vi "ObtainSMQueue.vi"(8 "ErrorArray In":errorcluster[](array[cluster]), 10 "BusNumber":u8) -> (0 "ErrorArray Out":errorcluster[](array[cluster]), 3 "QueRef":T1)   [LabVIEW 2014, in "Bus.lvlib" / "NISTBus.lvclass"]
uses:
  NISTBus.lvclass
  Framework/MsgQueue/TypeDef/QueRef.ctl
  Framework/MsgQueue/TypeDef/MsgQueue.ctl
  SMQueue.ctl
  <userlib>/NIST/NISTErrorLib/NISTErrorLib.lvlib
  Framework/TestFramework.lvlib
panel:
  out "Queue Name":string
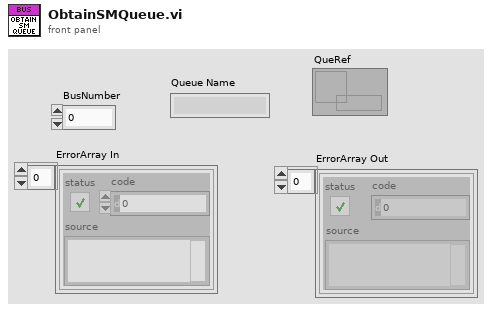
[diagram p1: front panel]
types:
  T1 = typedef "TestFramework.lvlib/QueRef.ctl" = refnum<queue>
  T2 = typedef "Bus.lvlib/NISTBus.lvclass/SMQueue.ctl" = cluster{"Msg":string, "Data":variant}
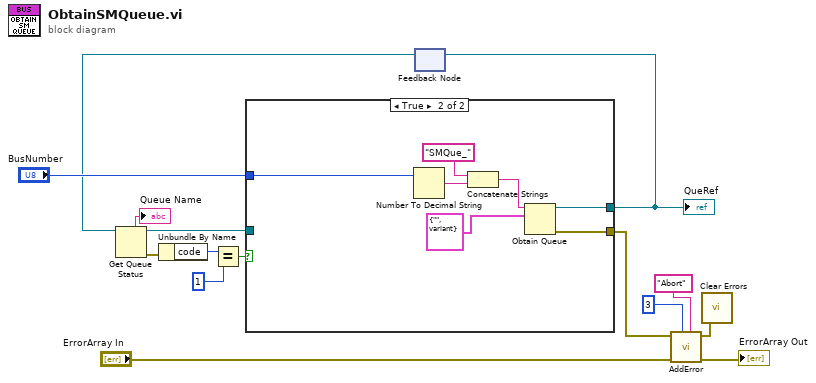
[diagram p0: block diagram]
diagram:
  n1 = feedback #1() -> (w2:refnum<queue>)  [unwired: 1 in]
  n2 = Get Queue Status(queue=w2) -> (queue out=w1:refnum<queue>, queue name=→"Queue Name":string, error out=w8:errorcluster)  [unwired: 2 in, 5 out]
  n3 = Unbundle By Name(w8) -> ("code"=w7:i32)
  n4 = Equal?(x=w7, y=1) -> (x = y?=w5:bool)
  n5 = case shown="True" w5 {
    tunnel: "BusNumber" -> [_ w21]
    tunnel: [w16 w19] -> w3
    tunnel: [_ w18] -> w12
    tunnel: w1 -> [w16 _]
    frame False {
    }
    frame True {
      n6 = Number To Decimal String(number=w21) -> (decimal integer string=w23:string)  [unwired: 1 in]
      n7 = Concatenate Strings("SMQue_" ("string"), w23) -> (w20:string)
      n8 = Obtain Queue(name (unnamed)=w20, element data type=T2 {"Msg"="", "Data"=variant} ("SMQueue")) -> (queue out=w19:refnum<queue>, error out=w18:errorcluster)  [unwired: 3 in, 1 out]
    }
  }
  "QueRef" <- w3
  n9 = feedback-in #1(w3) -> ()
  n10 = call <userlib>:"AddError.vi"("Severity"="Abort", "Priority"=u8 3, "ErrorArray"="ErrorArray In", "error in (no error)"=w12) -> ("ErrorArray"=→"ErrorArray Out":errorcluster[], "error out"=w9:errorcluster)  [unwired: 6 in]
  n11 = call <vilib>:"Clear Errors.vi"("error in (no error)"=w9) -> ()  [unwired: 5 in, 2 out]
